vi "Get Path Regex.vi"(8 "error in (no error)":errorcluster, 11 "StandardFileServe in":refnum<class "StandardFileServe.lvclass">) -> (0 "error out":errorcluster, 2 "Path Regex":string, 3 "StandardFileServe out":refnum<class "StandardFileServe.lvclass">)   [LabVIEW 2020, in "HTTP Server.lvlib" / "StandardFileServe.lvclass"]
uses:
  StandardFileServe.lvclass
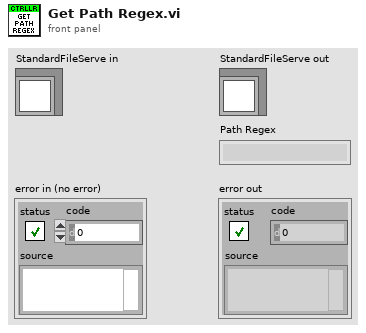
[diagram p1: front panel]
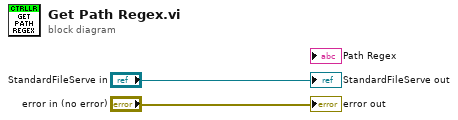
[diagram p0: block diagram]
diagram:
  "error out" <- "error in (no error)"
  "StandardFileServe out" <- "StandardFileServe in"
